vi "运维调试_采配水.vi"() -> ()   [LabVIEW 2016, in "PLC.lvlib"]
uses:
  PLC.lvlib
  control/switch.ctl
  <vilib>/Plasmionique/MB Master/MB_Master/MB_Master.lvclass
  <vilib>/Utility/miscctls.llb/LVPointTypeDef.ctl
  <vilib>/Plasmionique/MB Master/MB_Master_TCP/MB_Master_TCP.lvclass
  C:/Program Files (x86)/National Instruments/LabVIEW 2016/vi.lib/Plasmionique/MB Master/MB_Master/MB_Master.lvclass
  <vilib>/NI/Modbus Library/API/Wrapper/Create TCP Slave.vi
  <vilib>/NI/Modbus Library/API/slave/Modbus Slave.lvclass
  <vilib>/Plasmionique/MB Master/MB Master.lvlib
  <vilib>/NI/Modbus Library/API/Wrapper/API Main.lvlib
  <vilib>/Utility/config.llb/NI_LVConfig.lvlib
panel:
  in  "模拟量配置":bool
  out "过滤压力":sgl format="%#.4f"
  in  "三级过滤系统":bool
  out "配水泵计时":dbl
  out "氨氮水样池排液阀计时":dbl
  in  "M4":T1
  in  "V15":T1
  out "过滤出水阀计时":dbl
  out "过滤反冲洗阀计时":dbl
  out "过滤废水阀计时":dbl
  out "过滤回流阀计时":dbl
  out "过滤进样阀计时":dbl
  in  "V14-R":T1
  in  "V13-G":T1
  in  "V12":T1
  in  "V14-G":T1
  in  "V13-R":T1
  out "X8":bool caption="氨氮水样池液位开关_SL3"
  out "R122":i16 caption="氨氮水样池润洗时间"
  out "R123":i16 caption="过滤装置清洗时间"
  out "R121":i16 caption="过滤装置润洗时间"
  out "R120":i16 caption="加标回收配水时间"
  out "R116":i16 caption="储水时间设定"
  out "R115":i16 caption="清洗频次设定"
  out "R114":i16 caption="排液时间"
  out "R113":i16 caption="沉淀池清洗时间"
  out "R112":i16 caption="流通池清洗时间"
  out "R111":i16 caption="吹气时间"
  out "R110":i16 caption="外部管路清洗时间"
  out "R109":i16 caption="配水时间"
  out "R108":i16 caption="沉淀时间"
  out "R107":i16 caption="液位开关报警时间"
  out "R106":i16 caption="进样超时时间"
  out "R105":i16 caption="沉淀池润洗时间"
  out "R104":i16 caption="流通池润洗时间"
  out "沉淀池进样阀计时":dbl
  out "流通池进样阀计时":dbl
  in  "V3-R":T1
  in  "V3-G":T1
  out "状态":u16[](array[numeric])
  in  "更新程序":bool
  out "清洗次数":u16
  out "当前启动泵号":enum16{"1号泵", "2号泵"}(ring)
  in  "R117":u16(ring) caption="水箱储水水体" items=["自来水", "水样"]
  out "增压泵计时":dbl
  out "M2工作计时":dbl
  out "M1工作计时":dbl
  out "泵2反冲洗阀计时":dbl
  out "泵1反冲洗阀计时":dbl
  out "自来水出水阀计时":dbl
  out "进气阀计时":dbl
  out "流通池排液阀计时":dbl
  out "沉淀池排液阀计时":dbl
  out "沉淀池反冲洗阀计时":dbl
  out "流通池反冲洗阀计时":dbl
  out "泵2进样阀计时":dbl
  out "泵1进样阀计时":dbl
  in  "M3":T1
  in  "V11":T1
  in  "V10":T1
  in  "V2":T1
  in  "V1":T1
  in  "V7":T1
  in  "V6":T1
  out "X2":bool caption="进样水流开关_JY"
  out "采配水版本号":string
  out "通讯故障":bool
  in  "R102":u16(ring) caption="采水泵工作模式" items=["泵1单泵单管路", "泵2单泵单管路", "双泵双管路"]
  out "X7":bool caption="烟雾报警_YW"
  out "X6":bool caption="泵2过载报警_KM2"
  out "X5":bool caption="泵1过载报警_KM1"
  out "X4":bool caption="外部电源断电报警_DD1"
  out "X3":bool caption="水浸报警_SJ"
  out "X1":bool caption="沉淀池液位开关_YE2"
  out "X0":bool caption="流通池液位开关_YE1"
  out "集成报警信息":string
  out "R2":i16
  out "R1":i16
  out "多列列表框":i32(listbox)
  in  "V4":T1
  in  "V5":T1
  in  "V9":T1
  in  "V8":T1
  in  "M2":T1
  in  "M1":T1
  in  "返回":bool
  in  "参数设置":bool
  in  "单步启动":bool
  in  "启动":bool
  in  "停止":bool
  # "S"
  # "S"
  # "S"
  # "S"
  # "S"
  # "S"
  # "S"
  # "S"
  # "S"
  # "S"
  # "S"
  # "S"
  # "S"
  # "次"
  # "S"
  # "S"
  # "S"
  # "过滤压力："
  # "Mpa"
  # "单步计时："
  # "s"
  # "流程计时："
  # "s"
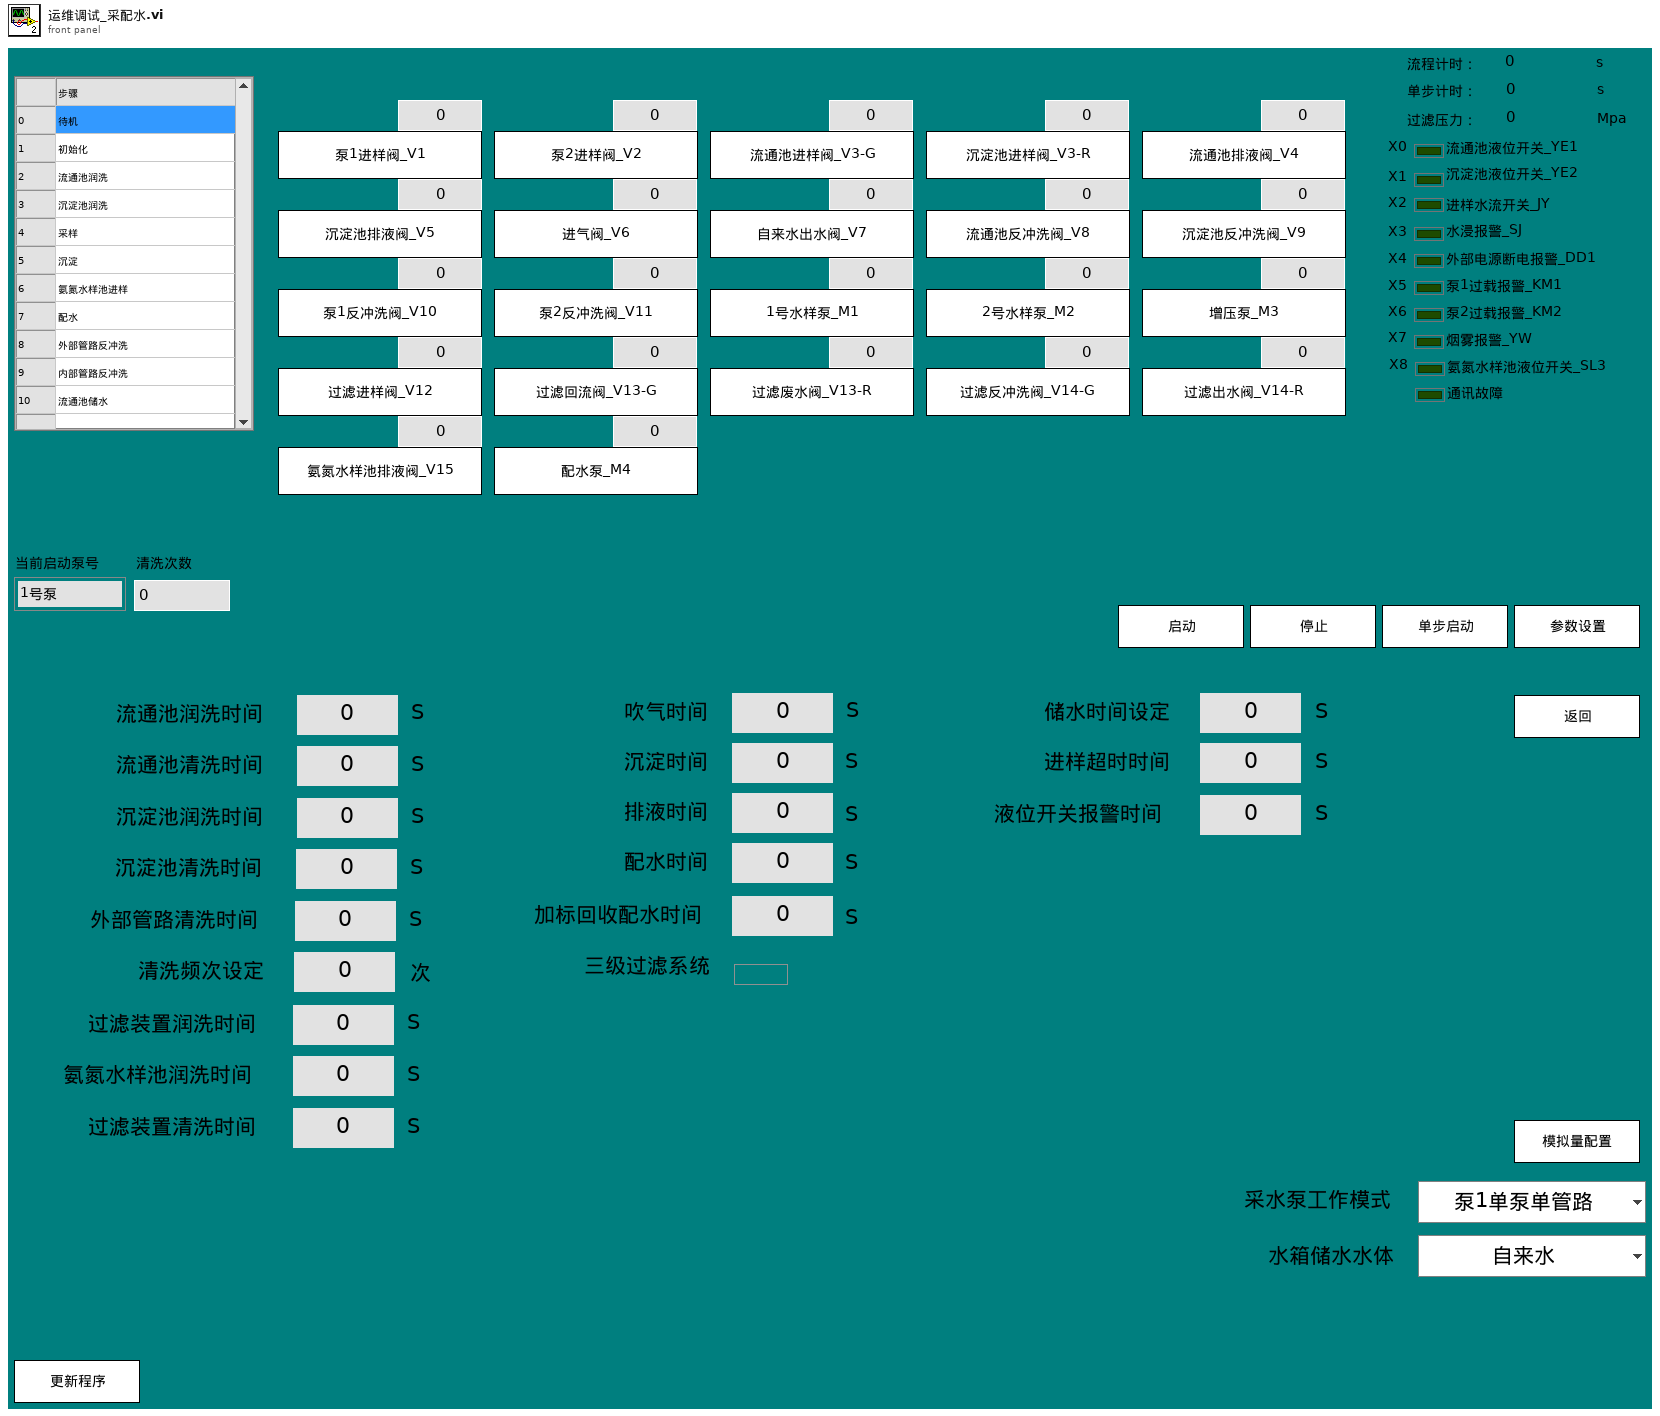
[diagram p1: front panel]
types:
  T1 = typedef "switch.ctl" = bool
  T2 = cluster{"R100":i16, "R101":i16, "R102":i16, "R103":i16, "R104":i16, "R105":i16, "R106":i16, "R107":i16, "R108":i16, "R109":i16, "R110":i16, "R111":i16, "R112":i16, "R113":i16, "R114":i16, "R115":i16, "R116":i16, "R117":i16, "R118":i16, "R119":i16, "R120":i16, "R121":i16, "R122":i16, "R123":i16}
  T3 = cluster{"R200":i16, "R201":i16, "R20 2":i16, "R20 3":i16, "R20 4":i16, "R20 5":i16, "R20 6":i16, "R20 7":i16, "R20 8":i16, "R20 9":i16, "R210":i16, "R211":i16, "R21 2":i16, "R21 3":i16, "R21 4":i16, "R21 5":i16, "R21 6":i16, "R21 7":i16, "R21 8":i16, "R21 9":i16, "R220":i16, "R221":i16, "R22 2":i16, "R22 3":i16, "R22 4":i16, "R22 5":i16, "R22 6":i16, "R22 7":i16, "R22 8":i16, "R22 9":i16, "R230":i16, "R231":i16}
  T4 = typedef "LVPointTypeDef.ctl" = cluster{"Horizontal":i16, "Vertical":i16}
  T5 = typedef "NI_LVConfig.lvlib/Config Data RefNum.ctl" = refnum<k1>
  T6 = cluster{"时间标识":timestamp, "设备":string, "日志信息":string}
  T7 = cluster{"R0":i16, "R1":i16, "R2":i16, "R3":i16, "R4":i16, "R5":i16, "R6":i16, "R7":i16, "R8":i16, "R9":i16, "R10":i16, "R11":i16, "R12":i16, "R13":i16, "R14":i16, "R15":i16, "R16":i16, "R17":i16, "R18":i16, "R19":i16, "R20":i16, "R21":i16, "R22":i16, "R23":i16, "R24":i16, "R25":i16, "R26":i16, "R27":i16, "R28":i16, "R29":i16, "R30":i16, "R31":i16, "R32":i16, "R33":i16, "R34":i16, "R35":i16, "R36":i16, "R37":i16, "R38":i16, "R39":i16}
  T8 = cluster{"seconds since 1Jan1904":timestamp, "table输入":string, string, "table输入":string}
  T9 = cluster{"时间标识":timestamp, "设备":string, "日志信息":string, "流程参数":string}
  T10 = cluster{"命令":string, cluster{"starting address":u16, "holding register value":u16}}
  T11 = cluster{"命令":string, "数据":cluster{"starting address":u16, "holding register value":u16}}
  T12 = cluster{"命令":string, "数据":cluster{"starting address":u16, "holding register values":u16[]}}
  T13 = cluster{"命令":string, "data":cluster{"starting address":u16, "coil values":bool[]}}
  T14 = cluster{"参数启用":cluster{"氨氮":bool, "总磷":bool, "总氮":bool, "多参数":bool, "CODMn":bool, "CODcr":bool, "超标留样":bool}}
  T15 = enum32{"Bad", "Idle", "Run top level", "Running"}
  T16 = cluster{"starting address":u16, "holding register values":u16[]}
  T17 = cluster{"starting address":u16, "holding register value":u16}
  T18 = cluster{"starting address":u16, "coil values":bool[]}
  T19 = cluster{"Registers[0]":u16, "Registers[1]":u16, "Registers[2]":u16, "Registers[3]":u16, "Registers[4]":u16, "Registers[5]":u16, "Registers[6]":u16, "Registers[7]":u16, "Registers[8]":u16, "Registers[9]":u16, "Registers[10]":u16, "Registers[11]":u16, "Registers[12]":u16, "Registers[13]":u16, "Registers[14]":u16, "Registers[15]":u16, "Registers[16]":u16, "Registers[17]":u16, "Registers[18]":u16, "Registers[19]":u16, "Registers[20]":u16, "Registers[21]":u16, "Registers[22]":u16, "Registers[23]":u16, "Registers[24]":u16, "Registers[25]":u16, "Registers[26]":u16, "Registers[27]":u16, "Registers[28]":u16, "Registers[29]":u16, "Registers[30]":u16, "Registers[31]":u16, "Registers[32]":u16, "Registers[33]":u16, "Registers[34]":u16, "Registers[35]":u16, "Registers[36]":u16, "Registers[37]":u16, "Registers[38]":u16, "Registers[39]":u16}
  T20 = cluster{"Registers[0]":u16, "Registers[1]":u16, "Registers[2]":u16, "Registers[3]":u16, "Registers[4]":u16, "Registers[5]":u16, "Registers[6]":u16, "Registers[7]":u16, "Registers[8]":u16, "Registers[9]":u16, "Registers[10]":u16, "Registers[11]":u16, "Registers[12]":u16, "Registers[13]":u16, "Registers[14]":u16, "Registers[15]":u16, "Registers[16]":u16, "Registers[17]":u16, "Registers[18]":u16, "Registers[19]":u16, "Registers[20]":u16, "Registers[21]":u16, "Registers[22]":u16, "Registers[23]":u16, "Registers[24]":u16, "Registers[25]":u16, "Registers[26]":u16, "Registers[27]":u16, "Registers[28]":u16, "Registers[29]":u16, "Registers[30]":u16, "Registers[31]":u16}
  T21 = cluster{"Registers[0]":u16, "Registers[1]":u16, "Registers[2]":u16, "Registers[3]":u16, "Registers[4]":u16, "Registers[5]":u16}
  T22 = cluster{"X0":dbl, "X1":dbl, "Y0":dbl, "Y1":dbl}[]
  T23 = cluster{"[0]":dbl, "[1]":dbl, "[2]":dbl, "[3]":dbl, "[4]":dbl, "[5]":dbl}
  T24 = cluster{"Registers[0]":u16, "Registers[1]":u16, "Registers[2]":u16, "Registers[3]":u16, "Registers[4]":u16, "Registers[5]":u16, "Registers[6]":u16, "Registers[7]":u16, "Registers[8]":u16, "Registers[9]":u16, "Registers[10]":u16, "Registers[11]":u16, "Registers[12]":u16, "Registers[13]":u16, "Registers[14]":u16, "Registers[15]":u16, "Registers[16]":u16, "Registers[17]":u16, "Registers[18]":u16, "Registers[19]":u16, "Registers[20]":u16, "Registers[21]":u16, "Registers[22]":u16, "Registers[23]":u16}
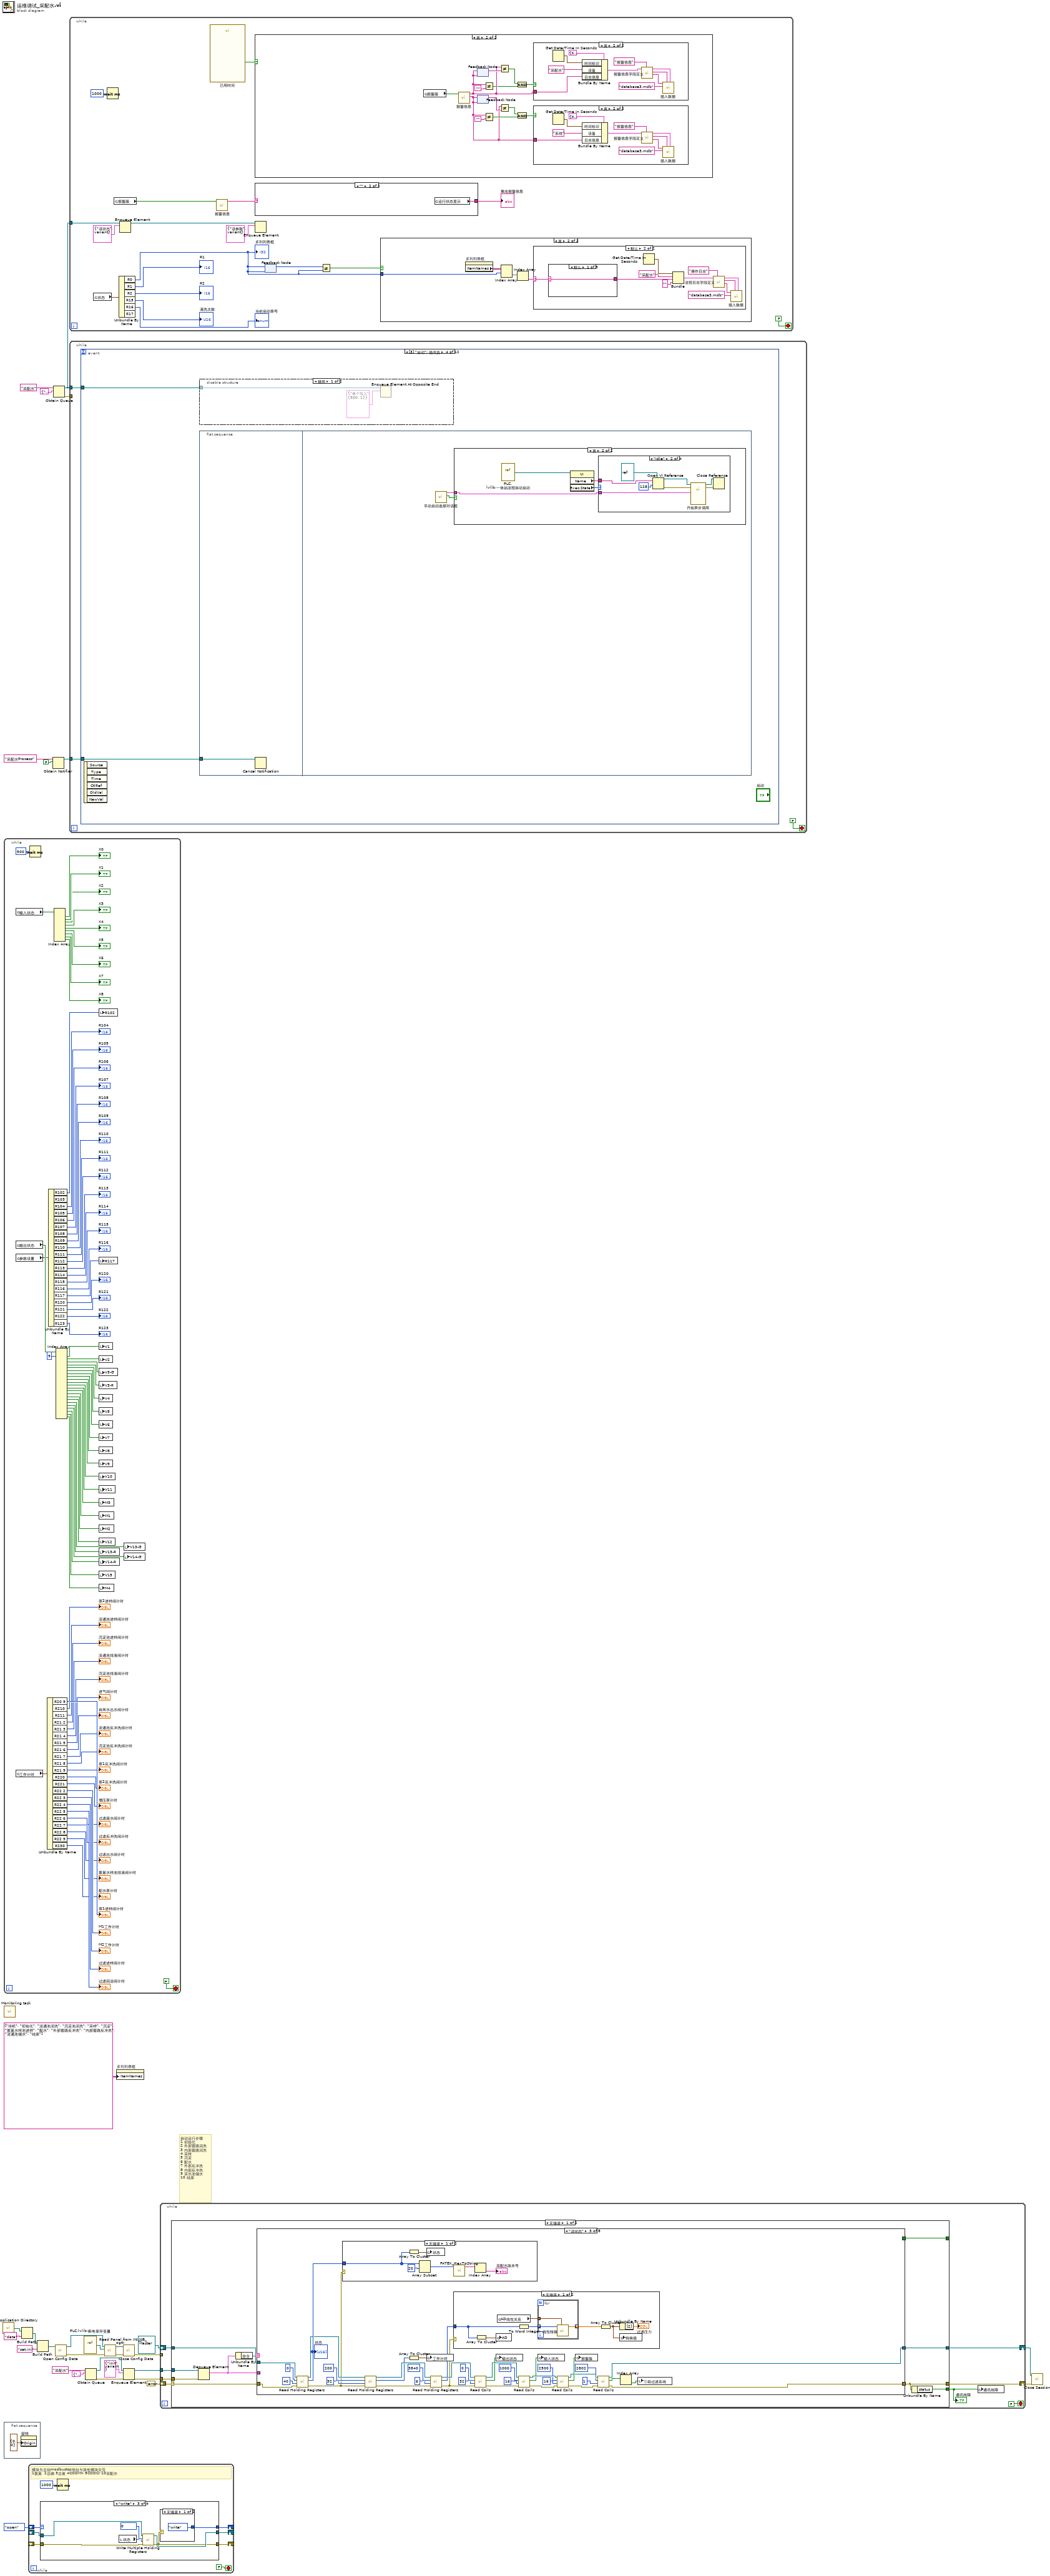
[diagram p0: block diagram]
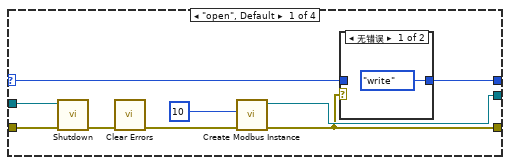
[diagram p2: hidden frame]
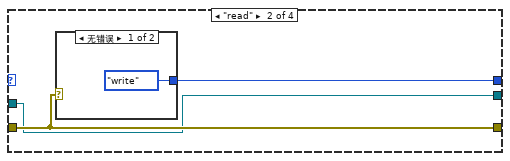
[diagram p4: hidden frame]
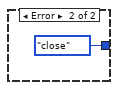
[diagram p5: hidden frame]
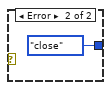
[diagram p6: hidden frame]
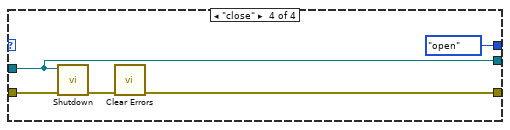
[diagram p7: hidden frame]
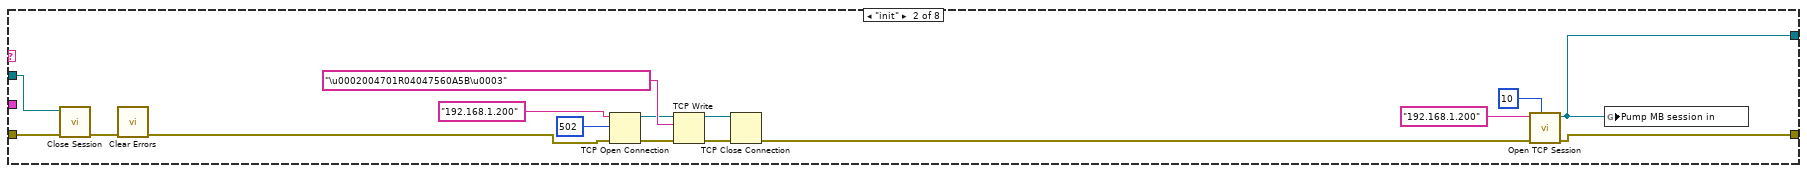
[diagram p9: hidden frame]
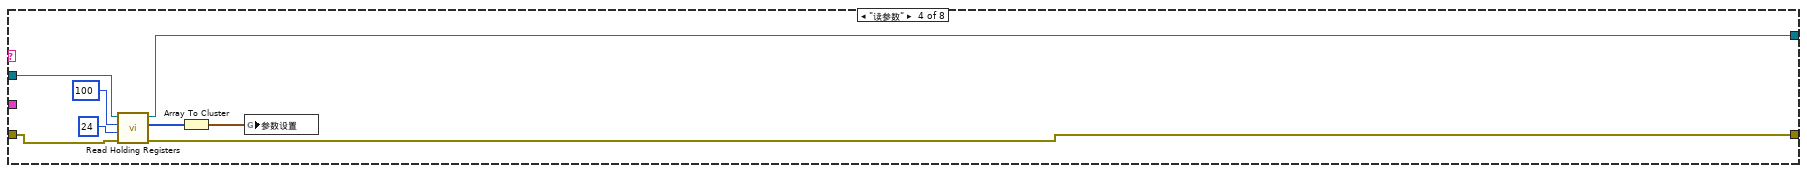
[diagram p12: hidden frame]
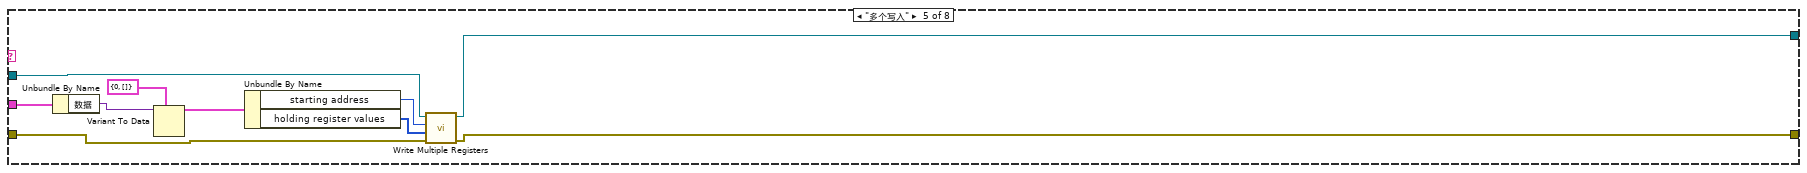
[diagram p13: hidden frame]
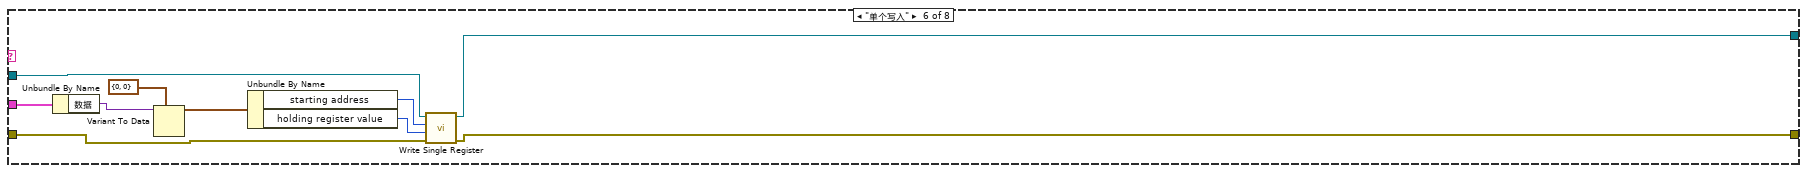
[diagram p14: hidden frame]
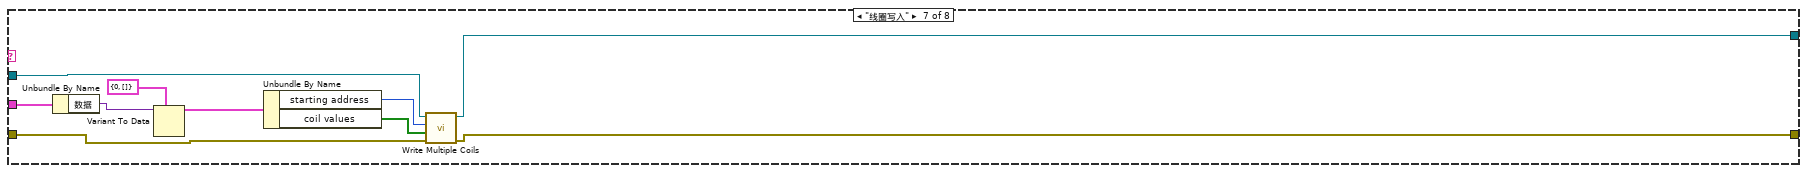
[diagram p15: hidden frame]
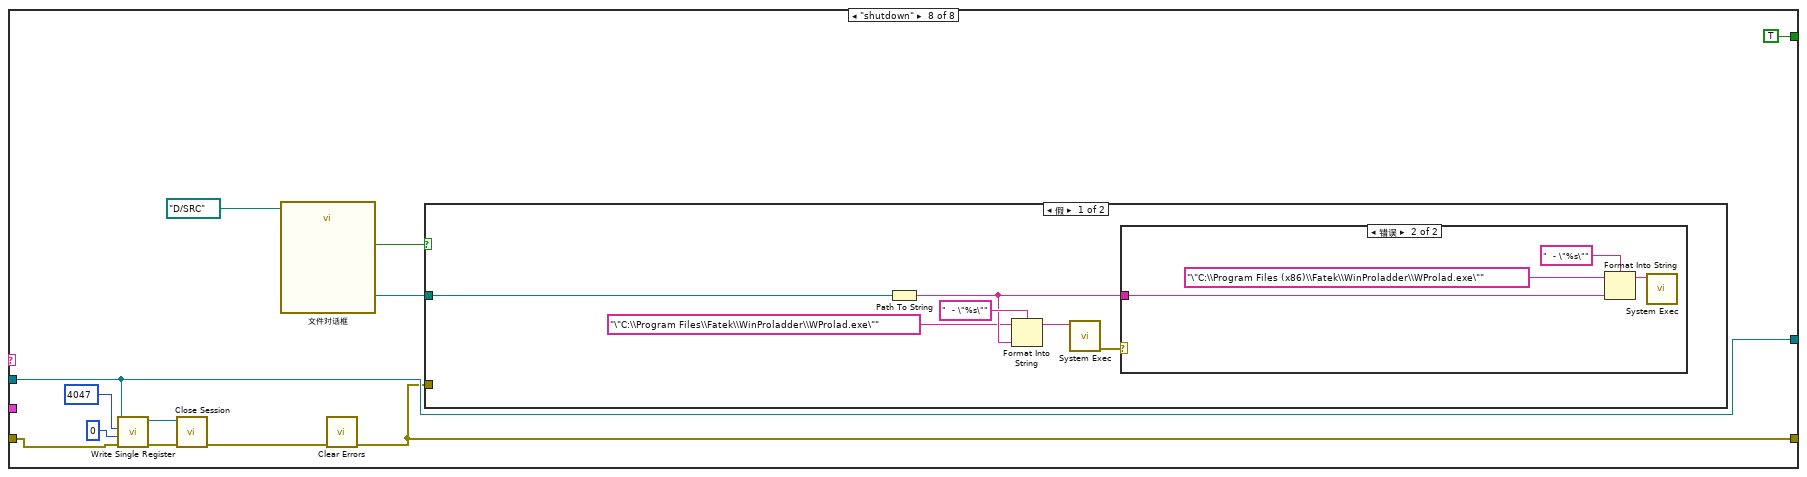
[diagram p16: hidden frame]
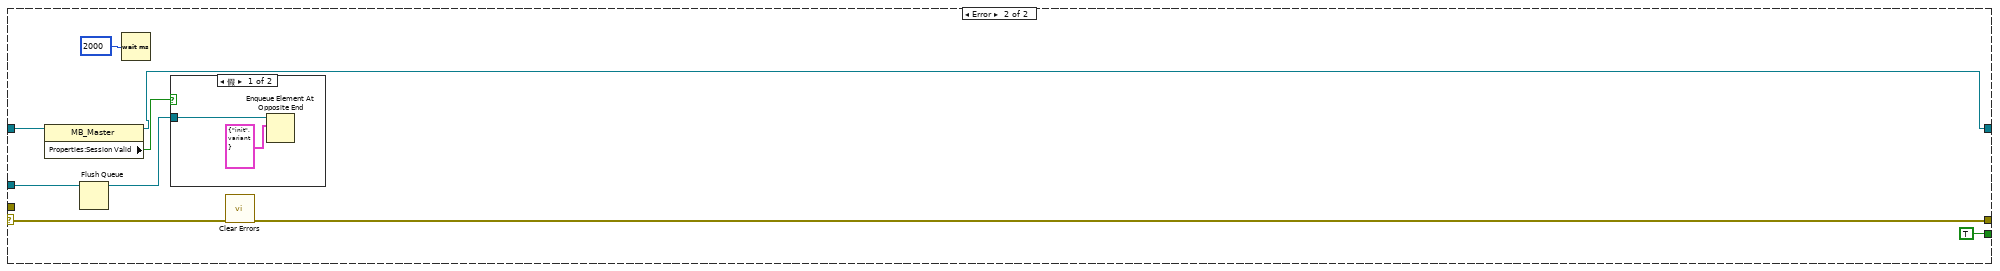
[diagram p19: hidden frame]
diagram:
  # "自动运行步骤\n1 初始化\n2 外部管路润洗\n3 内部管路润洗\n4 采样\n5 沉淀\n6 配水\n7 外部反冲洗\n8 内部反冲洗\n9 采水池储水\n10 结束"
  n1 = call <vilib>:"Application Directory.vi"() -> ("Application Directory"=w3:path)
  n2 = while {
    stop <- FALSE stop-if-true
    n3 = global read "采配水全局变量.vi" "输入状态"() -> (w93:bool[])
    n4 = global read "采配水全局变量.vi" "输出状态"() -> (w109:bool[])
    n5 = global read "采配水全局变量.vi" "参数设置"() -> (w66:T2)
    n6 = global read "采配水全局变量.vi" "工作计时"() -> (w82:T3)
    n7 = Wait (ms)(milliseconds to wait=u32 500 ("等待时间（毫秒）")) -> ()  [unwired: 1 out]
    n8 = Unbundle By Name(w82) -> ("R20 9"=→"泵1进样阀计时":i16, "R210"=→"泵2进样阀计时":i16, "R211"=→"流通池进样阀计时":i16, "R21 2"=→"沉淀池进样阀计时":i16, "R21 3"=→"流通池排液阀计时":i16, "R21 4"=→"沉淀池排液阀计时":i16, "R21 5"=→"进气阀计时":i16, "R21 6"=→"自来水出水阀计时":i16, "R21 7"=→"流通池反冲洗阀计时":i16, "R21 8"=→"沉淀池反冲洗阀计时":i16, "R21 9"=→"泵1反冲洗阀计时":i16, "R220"=→"泵2反冲洗阀计时":i16, "R221"=→"增压泵计时":i16, "R22 2"=→"M1工作计时":i16, "R22 3"=→"M2工作计时":i16, "R22 4"=→"过滤进样阀计时":i16, "R22 5"=→"过滤回流阀计时":i16, "R22 6"=→"过滤废水阀计时":i16, "R22 7"=→"过滤反冲洗阀计时":i16, "R22 8"=→"过滤出水阀计时":i16, "R22 9"=→"氨氮水样池排液阀计时":i16, "R230"=→"配水泵计时":i16)
    n9 = Unbundle By Name(w66) -> ("R102"=w65:i16, "R104"=→"R104":i16, "R105"=→"R105":i16, "R106"=→"R106":i16, "R107"=→"R107":i16, "R108"=→"R108":i16, "R109"=→"R109":i16, "R110"=→"R110":i16, "R111"=→"R111":i16, "R112"=→"R112":i16, "R113"=→"R113":i16, "R114"=→"R114":i16, "R115"=→"R115":i16, "R116"=→"R116":i16, "R117"=w51:i16, "R120"=→"R120":i16, "R121"=→"R121":i16, "R122"=→"R122":i16, "R123"=→"R123":i16)  [unwired: 1 out]
    n10 = Index Array(array=w93) -> (element #1=→"X0":bool, element #2=→"X1":bool, element #3=→"X2":bool, element #4=→"X3":bool, element #5=→"X4":bool, element #6=→"X5":bool, element #7=→"X6":bool, element #8=→"X7":bool, element #9=→"X8":bool)  [unwired: 9 in]
    n11 = Index Array(array=w109, index #1=9 ("索引")) -> (element #1=w107:bool, element #2=w106:bool, element #3=w105:bool, element #4=w104:bool, element #5=w103:bool, element #6=w102:bool, element #7=w101:bool, element #8=w100:bool, element #9=w83:bool, element #10=w84:bool, element #11=w99:bool, element #12=w98:bool, element #13=w97:bool, element #14=w96:bool, element #15=w95:bool, element #16=w47:bool, element #17=w46:bool, element #18=w45:bool, element #19=w44:bool, element #20=w43:bool, element #21=w42:bool, element #22=w41:bool)  [unwired: 21 in]
    n12 = local write "R102"(w65) -> ()
    n13 = local write "R117"(w51) -> ()
    n14 = local write "V1"(w107) -> ()
    n15 = local write "V2"(w106) -> ()
    n16 = local write "V3-G"(w105) -> ()
    n17 = local write "V3-R"(w104) -> ()
    n18 = local write "V4"(w103) -> ()
    n19 = local write "V5"(w102) -> ()
    n20 = local write "V6"(w101) -> ()
    n21 = local write "V7"(w100) -> ()
    n22 = local write "V8"(w83) -> ()
    n23 = local write "V9"(w84) -> ()
    n24 = local write "V10"(w99) -> ()
    n25 = local write "V11"(w98) -> ()
    n26 = local write "M3"(w97) -> ()
    n27 = local write "M1"(w96) -> ()
    n28 = local write "M2"(w95) -> ()
    n29 = local write "V12"(w47) -> ()
    n30 = local write "V13-R"(w45) -> ()
    n31 = local write "V14-R"(w43) -> ()
    n32 = local write "V15"(w42) -> ()
    n33 = local write "M4"(w41) -> ()
    n34 = local write "V13-G"(w46) -> ()
    n35 = local write "V14-G"(w44) -> ()
  }
  n36 = call "Monitoring task.vi"() -> ()  [unwired: 12 in]
  n37 = flat-sequence {
    frame #0 {
      n38 = property on="窗格" class="Pane"("Origin"=T4 {"Horizontal"=0, "Vertical"=0} ("原点")) -> ()  [unwired: 2 in, 2 out]
    }
  }
  n39 = Build Path(base path=w3, name or relative path="data" ("名称或相对路径")) -> (appended path=w5:path)
  n40 = while {
    shift-right: [w117] -> _
    shift-left: _ -> [w119]
    shift-right: [w116] -> _
    shift-left: _ -> [w118]
    shift-right: [w113] -> _
    shift-left: enum16{"open", "read", "write", "close"}."open" -> [w114]
    stop <- FALSE stop-if-true
    # "模块为主站modbustcp地址与其他模块交互\n1氨氮  2总磷 3总氮 4CODMn 5CODCr 10采配水"
    n41 = case shown="\"write\"" w114 {
      selector: w114 -> [w128 _ _ _]
      tunnel: w119 -> [w122 w131 w141 w147]
      tunnel: w118 -> [w121 w132 w140 w146]
      tunnel: [w125 w131 w138 w147] -> w117
      tunnel: [w124 w132 w137 w149] -> w116
      tunnel: [w127 w133 w142 enum16{"open", "read", "write", "close"}."open"] -> w113
      frame "open", Default {
        n42 = call-dynamic "Shutdown.vi"("error in"=w121, "Modbus slave in"=w122) -> ("error out"=w120:errorcluster)  [unwired: 9 in]
        n43 = call <vilib>:"Clear Errors.vi"("error in (no error)"=w120) -> ("error out"=w123:errorcluster)  [unwired: 5 in, 1 out]
        n44 = call-poly <vilib>:"Create Modbus Instance.vi"("error in"=w123, "port (502)"=u16 10) -> ("error out"=w124:errorcluster, "TCP slave instance"=w125:refnum<class "Modbus Slave.lvclass">)  [unwired: 8 in]
        n45 = case shown="无错误" w124 {
          tunnel: w128 -> [_ w130]
          tunnel: [enum16{"open", "read", "write", "close"}."write" w130] -> w127
          frame No Error {
          }
          frame Error {
          }
        }
      }
      frame "read" {
        n46 = case shown="无错误" w132 {
          tunnel: [enum16{"open", "read", "write", "close"}."write" enum16{"open", "read", "write", "close"}."close"] -> w133
          frame No Error {
          }
          frame Error {
          }
        }
      }
      frame "write" {
        n47 = local read "状态"() -> (w136:u16[])
        n48 = call-dynamic "Write Multiple Holding Registers.vi"("error in"=w140, "registers to write"=w136, "starting address"=u16 0, "Modbus slave in"=w141) -> ("error out"=w137:errorcluster, "Modbus slave out"=w138:refnum<class "Modbus Slave.lvclass">)  [unwired: 6 in]
        n49 = case shown="无错误" w137 {
          tunnel: [enum16{"open", "read", "write", "close"}."write" enum16{"open", "read", "write", "close"}."close"] -> w142
          frame No Error {
          }
          frame Error {
          }
        }
      }
      frame "close" {
        n50 = call-dynamic "Shutdown.vi"("error in"=w146, "Modbus slave in"=w147) -> ("error out"=w145:errorcluster)  [unwired: 9 in]
        n51 = call <vilib>:"Clear Errors.vi"("error in (no error)"=w145) -> ("error out"=w149:errorcluster)  [unwired: 5 in, 1 out]
      }
    }
    n52 = Wait (ms)(milliseconds to wait=u32 1000 ("等待时间（毫秒）")) -> ()  [unwired: 1 out]
  }
  n53 = Build Path(base path=w5, name or relative path="set.ini" ("名称或相对路径")) -> (appended path=w7:path)
  n54 = Obtain Notifier(name (unnamed)="采配水Process" ("名称（未命名）"), notification data type=FALSE) -> (notifier out=w24:refnum<notifier>)  [unwired: 2 in, 2 out]
  n55 = Obtain Queue(name (unnamed)="采配水" ("名称（未命名）"), element data type=cluster{"命令":string, "数据":variant} {"命令"="", "数据"=variant}) -> (queue out=w28:refnum<queue>, error out=w29:errorcluster)  [unwired: 3 in, 1 out]
  n56 = call <vilib>:"Open Config Data.vi"("configuration file path"=w7) -> ("error out"=w8:errorcluster, "refnum"=w2:T5)  [unwired: 8 in, 1 out]
  n57 = while {
    tunnel: w28 -> [w166]
    stop <- FALSE stop-if-true
    n58 = global read "采配水全局变量.vi" "状态"() -> (w164:T7)
    n59 = Wait (ms)(milliseconds to wait=u32 1000 ("等待时间（毫秒）")) -> ()  [unwired: 1 out]
    n60 = global read "采配水全局变量.vi" "报警簇"() -> (w160:bool[])
    n61 = Unbundle By Name(w164) -> ("R0"=w153:i16, "R1"=→"R1":i16, "R2"=→"R2":i16, "R15"=→"清洗次数":i16, "R16"=→"当前启动泵号":i16)  [unwired: 1 out]
    "多列列表框" <- w153
    n62 = Enqueue Element(queue=w166, element=cluster{"命令":string, "数据":variant} {"命令"="读状态", "数据"=variant} ("元素")) -> (queue out=w155:refnum<queue>)  [unwired: 2 in, 2 out]
    n63 = call "已用时间"() -> ("Time has Elapsed"=w158:bool)  [unwired: 12 in, 7 out]
    n64 = call "报警信息.vi"("报警簇"=w160) -> ("采配水报警信息"=w152:string)  [unwired: 9 in, 1 out]
    n65 = case shown="真" w158 {
      frame False {
      }
      frame True {
        n66 = global read "采配水全局变量.vi" "报警簇"() -> (w180:bool[])
        n67 = call "报警信息.vi"("报警簇"=w180) -> ("系统报警信息"=w169:string, "采配水报警信息"=w176:string)  [unwired: 9 in]
        n68 = feedback #1(w176) -> (w179:string)
        n69 = feedback-in #1(w176) -> ()
        n70 = feedback #2(w169) -> (w170:string)
        n71 = feedback-in #2(w169) -> ()
        n72 = Not Equal?(x=w176, y="") -> (x != y?=w174:bool)
        n73 = Not Equal?(x=w169, y="") -> (x != y?=w173:bool)
        n74 = Not Equal?(x=w176, y=w179) -> (x != y?=w178:bool)
        n75 = Not Equal?(x=w169, y=w170) -> (x != y?=w171:bool)
        n76 = And(x=w178, y=w174) -> (x .and. y?=w177:bool)
        n77 = And(x=w171, y=w173) -> (x .and. y?=w168:bool)
        n78 = case shown="真" w177 {
          tunnel: w176 -> [_ w191]
          frame False {
          }
          frame True {
            n79 = Get Date/Time In Seconds() -> (seconds since 1Jan1904=w193:timestamp)
            n80 = Bundle By Name(cluster=T6 {"时间标识"=timestamp(0 s since 1904-01-01), "设备"="", "日志信息"=""} ("data in"), "时间标识"=w193, "设备"="采配水", "日志信息"=w191) -> (w194:T6)
            n81 = call "报警信息字段定义.vi"("table输入"="报警信息", "data in"=w194) -> ("table输出"=w198:string, "columns"=w199:string[], "data out"=w200:T6)  [unwired: 7 in]
            n82 = call "插入数据.vi"("data"=w200, "columns"=w199, "database"="database3.mdb", "table"=w198) -> ()  [unwired: 7 in, 1 out]
          }
        }
        n83 = case shown="真" w168 {
          tunnel: w169 -> [_ w181]
          frame False {
          }
          frame True {
            n84 = Get Date/Time In Seconds() -> (seconds since 1Jan1904=w183:timestamp)
            n85 = Bundle By Name(cluster=T6 {"时间标识"=timestamp(0 s since 1904-01-01), "设备"="", "日志信息"=""} ("data in"), "时间标识"=w183, "设备"="系统", "日志信息"=w181) -> (w184:T6)
            n86 = call "报警信息字段定义.vi"("table输入"="报警信息", "data in"=w184) -> ("table输出"=w188:string, "columns"=w189:string[], "data out"=w190:T6)  [unwired: 7 in]
            n87 = call "插入数据.vi"("data"=w190, "columns"=w189, "database"="database3.mdb", "table"=w188) -> ()  [unwired: 7 in, 1 out]
          }
        }
      }
    }
    n88 = case shown="\"\"" w152 {
      selector: w152 -> [w201 _]
      tunnel: [w201 w202] -> w159
      frame Default {
      }
      frame "" {
        n89 = global read "采配水全局变量.vi" "运行状态显示"() -> (w202:string)
      }
    }
    "集成报警信息" <- w159
    n90 = Enqueue Element(queue=w155, element=cluster{"命令":string, "数据":variant} {"命令"="读参数", "数据"=variant} ("元素")) -> ()  [unwired: 2 in, 3 out]
    n91 = feedback-in #3(w153) -> ()
    n92 = feedback #3(w153) -> (w154:i16)
    n93 = Not Equal?(x=w154, y=w153) -> (x != y?=w161:bool)
    n94 = case shown="真" w161 {
      tunnel: w153 -> [_ w205]
      frame False {
      }
      frame True {
        n95 = property on="多列列表框" class="MCListbox (严格)"() -> ("ItemNames"=w206:string[][])  [unwired: 2 in, 2 out]
        n96 = Index Array(array=w206, index (row)=w205) -> (element=w204:string[])  [unwired: 1 in]
        n97 = Index Array(array=w204) -> (element=w203:string)  [unwired: 1 in]
        n98 = case shown="默认" w203 {
          selector: w203 -> [_ w208]
          frame "待机" {
          }
          frame Default {
            n99 = case shown="默认" w208 {
              selector: w208 -> [w218 _ _]
              tunnel: [w218 "-->>启动" "-->>结束"] -> w207
              frame Default {
              }
              frame "初始化" {
              }
              frame "结束" {
              }
            }
            n100 = Get Date/Time In Seconds() -> (seconds since 1Jan1904=w212:timestamp)
            n101 = Bundle("seconds since 1Jan1904"=w212, "table输入"="采配水", w207, "table输入"="") -> (w210:T8)  [unwired: 1 in]
            n102 = call "流程日志字段定义.vi"("table输入"="操作日志", "data in"=w210) -> ("table输出"=w215:string, "columns"=w216:string[], "data out"=w217:T9)  [unwired: 7 in]
            n103 = call "插入数据.vi"("data"=w217, "columns"=w216, "database"="database3.mdb", "table"=w215) -> ()  [unwired: 7 in, 1 out]
          }
        }
      }
    }
  }
  n104 = while {
    tunnel: w28 -> [w222]
    tunnel: w29 -> [_]
    tunnel: w24 -> [w221]
    stop <- FALSE stop-if-true
    n105 = event shown="[3] \"启动\": 值改变" {
      selector: _ -> [_ _ _ _ _ _ _ _ _ _ _ _]
      dyn-events: _ -> [_ _ _ _ _ _ _ _ _ _ _ _]
      timeout: _ -> [_ _ _ _ _ _ _ _ _ _ _ _]
      tunnel: w222 -> [_ _ w226 w229 w251 w259 _ _ _ w315 w318 w325]
      tunnel: w221 -> [_ _ w225 w228 _ _ _ _ _ _ _ _]
      event Timeout {
        n106 = event-data() -> ()  [unwired: 1 in, 3 out]
      }
      event "模拟量配置": Value Change {
        n107 = event-data() -> ()  [unwired: 1 in, 6 out]
        n108 = call "模拟量设置窗口.vi"() -> ()  [unwired: 12 in]
      }
      event "停止": Value Change {
        n109 = event-data() -> ()  [unwired: 1 in, 6 out]
        n110 = Send Notification(notification=TRUE ("通知"), notifier=w225) -> ()  [unwired: 1 in, 2 out]
        n111 = Enqueue Element At Opposite End(queue=w226, element=T10 {"命令"="单个写入", {"starting address"=300, "holding register value"=2}} ("元素")) -> ()  [unwired: 2 in, 3 out]
      }
      event "启动": Value Change {
        n112 = event-data() -> ()  [unwired: 1 in, 6 out]
        n113 = disable-structure shown="禁用" {
          disable-tunnel: w229 -> [w247 _]
          frame Disabled {
            n114 = Enqueue Element At Opposite End(queue=w247, element=T10 {"命令"="单个写入", {"starting address"=300, "holding register value"=1}} ("元素")) -> ()  [unwired: 2 in, 3 out]
          }
          frame Enabled {
          }
        }
        n115 = flat-sequence {
          tunnel: w228 -> [w230]
          frame #0 {
            n116 = Cancel Notification(0:w230) -> ()  [unwired: 1 in, 3 out]
          }
          frame #1 {
            n117 = call "手动启动选择对话框.vi"() -> ("确定"=w232:bool, "输出簇"=w231:T14)  [unwired: 10 in]
            n118 = case shown="真" w232 {
              tunnel: w231 -> [_ w233]
              frame False {
              }
              frame True {
                n119 = vi-ref "PLC.lvlib:一体站流程自动启动.vi"() -> (w236:refnum<vi>)
                n120 = property class="VI"(reference=w236) -> ("Name"=w235:string, "Exec.State"=w234:T15)  [unwired: 1 in, 2 out]
                n121 = case shown="\"Idle\"" w234 {
                  tunnel: w235 -> [_ w244 _ _]
                  tunnel: w233 -> [_ w238 _ _]
                  frame "Bad", Default {
                  }
                  frame "Idle" {
                    n122 = Open VI Reference(type specifier VI Refnum (for type only)=refnum<vi> refnum, vi path=w244, options=128 ("选项")) -> (vi reference=w242:refnum<vi>, error out=w240:errorcluster)  [unwired: 3 in]
                    n123 = call-by-ref "开始异步调用"(reference=w242, error in=w240, "参数"=w238) -> (reference out=w241:refnum<vi>, error out=w239:errorcluster)  [unwired: 11 in]
                    n124 = Close Reference(reference=w241, error in (no error)=w239) -> ()  [unwired: 1 out]
                  }
                  frame "Run top level" {
                  }
                  frame "Running" {
                    n125 = One Button Dialog(message="流程已启动，无需重复启动！" ("消息")) -> ()  [unwired: 1 in, 1 out]
                  }
                }
              }
            }
          }
        }
      }
      event "单步启动": Value Change {
        n126 = event-data() -> ()  [unwired: 1 in, 6 out]
        n127 = call "单步启动对话框.vi"() -> ("单步启动步骤输出"=w248:u16)  [unwired: 11 in]
        n128 = Bundle By Name(cluster=T11 {"命令"="单个写入", "数据"={"starting address"=301, "holding register value"=0}} ("元素"), "数据.holding register value"=w248) -> (w249:T11)
        n129 = Enqueue Element At Opposite End(queue=w251, element=w249) -> ()  [unwired: 2 in, 3 out]
      }
      event "R104", "R117", "R105", "R106", "R107", "R108", "R109", "R110", "R111", "R112", "R113", "R114", "R115", "R116", "R102", "R120", "R121", "R123", "R122": Value Change {
        n130 = event-data() -> ()  [unwired: 1 in, 6 out]
        n131 = local read "R104"() -> (w277:i16)
        n132 = local read "R105"() -> (w276:i16)
        n133 = local read "R106"() -> (w275:i16)
        n134 = local read "R107"() -> (w274:i16)
        n135 = local read "R108"() -> (w273:i16)
        n136 = local read "R109"() -> (w272:i16)
        n137 = local read "R110"() -> (w271:i16)
        n138 = local read "R111"() -> (w270:i16)
        n139 = local read "R112"() -> (w269:i16)
        n140 = local read "R113"() -> (w268:i16)
        n141 = local read "R114"() -> (w267:i16)
        n142 = local read "R115"() -> (w266:i16)
        n143 = local read "R116"() -> (w265:i16)
        n144 = Build Array("R102", u16 0 ("元素"), w277, w276, w275, w274, w273, w272, w271, w270, w269, w268, w267, w266, w265, "R117") -> (w278:u16[])
        n145 = local read "R120"() -> (w257:i16)
        n146 = local read "R121"() -> (w255:i16)
        n147 = local read "R122"() -> (w254:i16)
        n148 = local read "R123"() -> (w253:i16)
        n149 = Build Array(w257, w255, w254, w253) -> (w256:i16[])
        n150 = Bundle By Name(cluster=T12 {"命令"="多个写入", "数据"={"starting address"=0, "holding register values"=[]}} ("元素"), "数据.starting address"=u16 102, "数据.holding register values"=w278) -> (w280:T12)
        n151 = Flush Queue(queue=w259) -> (queue out=w252:refnum<queue>)  [unwired: 1 in, 2 out]
        n152 = Bundle By Name(cluster=T12 {"命令"="多个写入", "数据"={"starting address"=0, "holding register values"=[]}} ("元素"), "数据.starting address"=u16 120, "数据.holding register values"=w256) -> (w262:T12)
        n153 = Enqueue Element At Opposite End(queue=w252, element=w280) -> (error out=w258:errorcluster)  [unwired: 2 in, 2 out]
        n154 = Enqueue Element At Opposite End(queue=w252, element=w262, error in (no error)=w258) -> ()  [unwired: 1 in, 3 out]
      }
      event "R104", "R105", "R106", "R107", "R108", "R109", "R110", "R111", "R112", "R113", "R114", "R115", "R116", "R120", "R122", "R123", "R121": Mouse Down {
        n155 = event-data() -> ("CtlRef"=w286:refnum<vi>)  [unwired: 1 in, 7 out]
        n156 = property class="DigNum (严格)"(reference=w286) -> (reference out=w284:refnum<vi>, "Value"=w285:i16)  [unwired: 1 in, 1 out]
        n157 = call "数字键盘.vi"("OldNumber"=w285) -> ("NewNumber"=w283:sgl)
        n158 = property class="DigNum (严格)"(reference=w284, "Val(Sgnl)"=w283) -> ()  [unwired: 1 in, 2 out]
      }
      event "参数设置": Value Change {
        n159 = event-data() -> ()  [unwired: 1 in, 6 out]
        n160 = property on="窗格" class="Pane"("Origin"=T4 {"Horizontal"=0, "Vertical"=628} ("原点")) -> ()  [unwired: 2 in, 2 out]
      }
      event "返回": Value Change {
        n161 = event-data() -> ()  [unwired: 1 in, 6 out]
        n162 = property on="窗格" class="Pane"("Origin"=T4 {"Horizontal"=0, "Vertical"=0} ("原点")) -> ()  [unwired: 2 in, 2 out]
      }
      event Value Change {
        n163 = event-data() -> ()  [unwired: 1 in, 6 out]
        n164 = Build Array("V1", "V2", "V3-G", "V3-R", "V4", "V5", "V6", "V7", "V8", "V9", "V10", "V11", "M3", "M1", "M2", "V12", "V13-G", "V13-R", "V14-G", "V14-R", "V15", "M4") -> (w312:T1[])
        n165 = Bundle By Name(cluster=T13 {"命令"="线圈写入", "data"={"starting address"=2409, "coil values"=[]}} ("元素"), "data.coil values"=w312) -> (w313:T13)
        n166 = Flush Queue(queue=w315) -> (queue out=w289:refnum<queue>)  [unwired: 1 in, 2 out]
        n167 = Enqueue Element At Opposite End(queue=w289, element=w313) -> ()  [unwired: 2 in, 3 out]
      }
      event "三级过滤系统": Value Change {
        n168 = event-data() -> ()  [unwired: 1 in, 6 out]
        n169 = Build Array("三级过滤系统") -> (w316:bool[])
        n170 = Bundle By Name(cluster=T13 {"命令"="线圈写入", "data"={"starting address"=2802, "coil values"=[]}} ("元素"), "data.coil values"=w316) -> (w320:T13)
        n171 = Flush Queue(queue=w318) -> (queue out=w319:refnum<queue>)  [unwired: 1 in, 2 out]
        n172 = Enqueue Element At Opposite End(queue=w319, element=w320) -> ()  [unwired: 2 in, 3 out]
      }
      event "更新程序": Value Change {
        n173 = event-data() -> ("NewVal"=w322:bool)  [unwired: 1 in, 5 out]
        n174 = case shown="真" w322 {
          tunnel: [cluster{"命令":string, "数据":variant} {"命令"="init", "数据"=variant} ("元素") w329] -> w324
          frame False {
          }
          frame True {
            n175 = Two Button Dialog(message="警告，非专业人士请勿进行此操作！！！\n请确认是否继续？" ("消息")) -> (T button?=w328:bool)  [unwired: 2 in]
            n176 = case shown="假" w328 {
              tunnel: [_ cluster{"命令":string, "数据":variant} {"命令"="shutdown", "数据"=variant} ("元素")] -> w329
              frame False {
                n177 = local write "更新程序"(FALSE ("释放串口")) -> ()
              }
              frame True {
              }
            }
          }
        }
        n178 = Flush Queue(queue=w325) -> (queue out=w323:refnum<queue>)  [unwired: 1 in, 2 out]
        n179 = Enqueue Element(queue=w323, element=w324) -> ()  [unwired: 2 in, 3 out]
      }
    }
  }
  n180 = vi-ref "PLC.lvlib:断电保存变量.vi"() -> (w9:refnum<vi>)
  n181 = Obtain Queue(name (unnamed)="采配水" ("名称（未命名）"), element data type=cluster{"命令":string, "数据":variant} {"命令"="", "数据"=variant}) -> (queue out=w21:refnum<queue>, error out=w20:errorcluster)  [unwired: 3 in, 1 out]
  n182 = call <userlib>:"Read Panel from INI__ogtk.vi"("error in (no error)"=w8, "VI ref"=w9, "refnum"=w2) -> ("error out"=w11:errorcluster, "refnum out"=w10:T5)  [unwired: 7 in]
  n183 = property on="多列列表框" class="MCListbox (严格)"("ItemNames"=string[][] [["待机"], ["初始化"], ["流通池润洗"], ["沉淀池润洗"], ["采样"], ["沉淀"], ["氨氮水样池进样"], ["配水"], ["外部管路反冲洗"], ["内部管路反冲洗"], ["流通池储水"], ["结束"]] ("项名")) -> ()  [unwired: 2 in, 2 out]
  n184 = call <vilib>:"Close Config Data.vi"("error in (no error)"=w11, "refnum"=w10) -> ("error out"=w1:errorcluster)  [unwired: 8 in, 1 out]
  n185 = Enqueue Element(queue=w21, element=cluster{"命令":string, "数据":variant} {"命令"="init", "数据"=variant} ("元素"), error in (no error)=w20) -> (queue out=w16:refnum<queue>, error out=w18:errorcluster)  [unwired: 1 in, 1 out]
  n186 = while {
    tunnel: w16 -> [w337]
    tunnel: w18 -> [w336]
    shift-right: [w339] -> w15
    shift-left: refnum<class "MB_Master.lvclass"> refnum ("MB session out") -> [w338]
    shift-right: [w334] -> w12
    shift-left: errorcluster {"status"=FALSE, "code"=0, "source"=""} ("error out") -> [w333]
    tunnel: w1 -> [_]
    stop <- FALSE stop-if-true
    n187 = case shown="无错误" w333 {
      selector: w333 -> [w347 w487]
      tunnel: [w349 w484] -> w339
      tunnel: w338 -> [w348 w485]
      tunnel: [w341 w488] -> w334
      tunnel: w337 -> [w344 w491]
      tunnel: w336 -> [w343 _]
      tunnel: [w345 _] -> _
      tunnel: [w340 TRUE ("status")] -> w332
      frame No Error {
        n188 = Dequeue Element(queue=w344, error in (no error)=w343) -> (element=w342:cluster{"命令":string, "数据":variant})  [unwired: 1 in, 3 out]
        n189 = Unbundle By Name(w342) -> ("命令"=w346:string)
        n190 = case shown="\"读状态\"" w346 {
          tunnel: [w351 w352 w376 w425 w437 w447 w457 w470] -> w349
          tunnel: w348 -> [w351 w365 w403 w430 w440 w450 w460 w470]
          tunnel: [w350 w362 w372 w424 w438 w448 w458 w461] -> w341
          tunnel: w347 -> [w350 w367 w406 w429 w439 w449 w459 w466]
          tunnel: [_ _ _ _ _ _ _ TRUE] -> w345
          tunnel: w342 -> [_ _ _ _ w436 w446 w456 _]
          frame "idle", Default {
          }
          frame "init" {
            n191 = call-dynamic "Close Session.vi"("error in (no error)"=w367, "MB session in"=w365) -> ("error out"=w366:errorcluster)  [unwired: 9 in]
            n192 = call <vilib>:"Clear Errors.vi"("error in (no error)"=w366) -> ("error out"=w354:errorcluster)  [unwired: 5 in, 1 out]
            n193 = TCP Open Connection(address="192.168.1.200" ("IP Address"), remote port or service name=u16 502 ("远程端口或服务名称"), error in (no error)=w354) -> (connection ID=w356:refnum<k5>, error out=w355:errorcluster)  [unwired: 2 in]
            n194 = TCP Write(connection ID=w356, data in="\u0002004701R04047560A5B\u0003" ("写入缓冲区"), error in (no error)=w355) -> (connection ID out=w357:refnum<k5>, error out=w358:errorcluster)  [unwired: 1 in, 1 out]
            n195 = TCP Close Connection(connection ID=w357, error in (no error)=w358) -> (error out=w353:errorcluster)  [unwired: 1 in, 1 out]
            n196 = call <vilib>:"Open TCP Session.vi"("Slave ID (255)"=u8 10, "error in (no error)"=w353, "IP Address"="192.168.1.200") -> ("error out"=w362:errorcluster, "MB_TCP session"=w352:refnum<class "MB_Master_TCP.lvclass">)  [unwired: 7 in]
            n197 = global write "采配水全局变量.vi" "Pump MB session in"(w352) -> ()
          }
          frame "读状态" {
            n198 = call <vilib>:"Read Holding Registers.vi"("error in (no error)"=w406, "quantity"=u16 40 ("number of holding registers"), "starting address"=u16 0, "MB session in"=w403) -> ("error out"=w369:errorcluster, "Registers"=w385:u16[], "MB session out"=w384:refnum<class "MB_Master.lvclass">)  [unwired: 5 in]
            "状态" <- w385
            n199 = case shown="无错误" w369 {
              tunnel: w385 -> [w418 _]
              frame No Error {
                n200 = Array To Cluster(array=w418) -> (cluster=w417:T19)
                n201 = Array Subset(array=w418, index=20 ("索引")) -> (w421:u16[])  [unwired: 1 in]
                n202 = global write "采配水全局变量.vi" "状态"(w417) -> ()
                n203 = call "FATEK_HexToString.vi"("数组"=w421) -> ("STRING"=w420:string[])  [unwired: 10 in]
                n204 = Index Array(array=w420) -> (element=→"采配水版本号":string)  [unwired: 1 in]
              }
              frame Error {
              }
            }
            n205 = call <vilib>:"Read Holding Registers.vi"("error in (no error)"=w369, "quantity"=u16 32, "starting address"=u16 200, "MB session in"=w384) -> ("error out"=w383:errorcluster, "Registers"=w379:u16[], "MB session out"=w382:refnum<class "MB_Master.lvclass">)  [unwired: 5 in]
            n206 = Array To Cluster(array=w379) -> (cluster=w378:T20)
            n207 = global write "采配水全局变量.vi" "工作计时"(w378) -> ()
            n208 = call <vilib>:"Read Holding Registers.vi"("error in (no error)"=w383, "quantity"=u16 6 ("number of holding registers"), "starting address"=u16 3840, "MB session in"=w382) -> ("error out"=w368:errorcluster, "Registers"=w386:u16[], "MB session out"=w400:refnum<class "MB_Master.lvclass">)  [unwired: 5 in]
            n209 = case shown="无错误" w368 {
              tunnel: w386 -> [w412 _]
              frame No Error {
                n210 = Array To Cluster(array=w412) -> (cluster=w413:T21)
                n211 = global write "采配水全局变量.vi" "AD"(w413) -> ()
                n212 = global read "断电保存变量.vi" "AD线性关系"() -> (w411:T22)
                n213 = To Word Integer(number=w412) -> (16bit integer=w410:i16[])
                n214 = for {
                  tunnel: w411 -> [w416] mode=indexing
                  tunnel: w410 -> [w415] mode=indexing
                  tunnel: [w414] -> w409 mode=indexing
                  n215 = call "线性转换.vi"("线性关系"=w416, "input"=w415) -> ("output"=w414:dbl)  [unwired: 9 in]
                }
                n216 = Array To Cluster(array=w409) -> (cluster=w408:T23)
                n217 = Unbundle By Name(w408) -> ("[2]"=→"过滤压力":dbl)
                n218 = global write "采配水全局变量.vi" "转换值"(w408) -> ()
              }
              frame Error {
              }
            }
            n219 = call <vilib>:"Read Coils.vi"("error in (no error)"=w368, "quantity"=u16 32 ("number of coils"), "starting address"=u16 0, "MB session in"=w400) -> ("error out"=w396:errorcluster, "Coils"=w387:bool[], "MB session out"=w397:refnum<class "MB_Master.lvclass">)  [unwired: 5 in]
            n220 = global write "采配水全局变量.vi" "输出状态"(w387) -> ()
            n221 = call <vilib>:"Read Coils.vi"("error in (no error)"=w396, "quantity"=u16 16 ("number of coils"), "starting address"=u16 1000, "MB session in"=w397) -> ("error out"=w392:errorcluster, "Coils"=w388:bool[], "MB session out"=w393:refnum<class "MB_Master.lvclass">)  [unwired: 5 in]
            n222 = global write "采配水全局变量.vi" "输入状态"(w388) -> ()
            n223 = call <vilib>:"Read Coils.vi"("error in (no error)"=w392, "quantity"=u16 16 ("number of coils"), "starting address"=u16 2500, "MB session in"=w393) -> ("error out"=w375:errorcluster, "Coils"=w389:bool[], "MB session out"=w377:refnum<class "MB_Master.lvclass">)  [unwired: 5 in]
            n224 = global write "采配水全局变量.vi" "报警簇"(w389) -> ()
            n225 = call <vilib>:"Read Coils.vi"("error in (no error)"=w375, "quantity"=u16 1 ("starting address"), "starting address"=u16 2802, "MB session in"=w377) -> ("error out"=w372:errorcluster, "Coils"=w371:bool[], "MB session out"=w376:refnum<class "MB_Master.lvclass">)  [unwired: 5 in]
            n226 = Index Array(array=w371) -> (element=w370:bool)  [unwired: 1 in]
            n227 = local write "三级过滤系统"(w370) -> ()
          }
          frame "读参数" {
            n228 = call <vilib>:"Read Holding Registers.vi"("error in (no error)"=w429, "quantity"=u16 24 ("number of holding registers"), "starting address"=u16 100, "MB session in"=w430) -> ("error out"=w424:errorcluster, "Registers"=w426:u16[], "MB session out"=w425:refnum<class "MB_Master.lvclass">)  [unwired: 5 in]
            n229 = Array To Cluster(array=w426) -> (cluster=w423:T24)
            n230 = global write "采配水全局变量.vi" "参数设置"(w423) -> ()
          }
          frame "多个写入" {
            n231 = Unbundle By Name(w436) -> ("数据"=w435:variant)
            n232 = Variant To Data(type=T16 {"starting address"=0, "holding register values"=[]}, Variant=w435) -> (data=w433:T16)  [unwired: 1 in, 1 out]
            n233 = Unbundle By Name(w433) -> ("starting address"=w432:u16, "holding register values"=w431:u16[])
            n234 = call <vilib>:"Write Multiple Registers.vi"("error in (no error)"=w439, "values"=w431, "starting address"=w432, "MB session in"=w440) -> ("error out"=w438:errorcluster, "MB session out"=w437:refnum<class "MB_Master.lvclass">)  [unwired: 6 in]
          }
          frame "单个写入" {
            n235 = Unbundle By Name(w446) -> ("数据"=w445:variant)
            n236 = Variant To Data(type=T17 {"starting address"=0, "holding register value"=0}, Variant=w445) -> (data=w443:T17)  [unwired: 1 in, 1 out]
            n237 = Unbundle By Name(w443) -> ("starting address"=w442:u16, "holding register value"=w441:u16)
            n238 = call <vilib>:"Write Single Register.vi"("error in (no error)"=w449, "value"=w441, "address"=w442, "MB session in"=w450) -> ("error out"=w448:errorcluster, "MB session out"=w447:refnum<class "MB_Master.lvclass">)  [unwired: 6 in]
          }
          frame "线圈写入" {
            n239 = Unbundle By Name(w456) -> ("数据"=w455:variant)
            n240 = Variant To Data(type=T18 {"starting address"=0, "coil values"=[]}, Variant=w455) -> (data=w453:T18)  [unwired: 1 in, 1 out]
            n241 = Unbundle By Name(w453) -> ("starting address"=w452:u16, "coil values"=w451:bool[])
            n242 = call <vilib>:"Write Multiple Coils.vi"("error in (no error)"=w459, "values"=w451, "starting address"=w452, "MB session in"=w460) -> ("error out"=w458:errorcluster, "MB session out"=w457:refnum<class "MB_Master.lvclass">)  [unwired: 6 in]
          }
          frame "shutdown" {
            n243 = call <vilib>:"Write Single Register.vi"("error in (no error)"=w466, "value"=u16 0, "address"=u16 4047, "MB session in"=w470) -> ("error out"=w465:errorcluster, "MB session out"=w469:refnum<class "MB_Master.lvclass">)  [unwired: 6 in]
            n244 = call-dynamic "Close Session.vi"("error in (no error)"=w465, "MB session in"=w469) -> ("error out"=w471:errorcluster)  [unwired: 9 in]
            n245 = call "文件对话框"("start path"=path "D:/SRC") -> ("selected path"=w464:path, "cancelled"=w462:bool)  [unwired: 11 in, 2 out]
            n246 = call <vilib>:"Clear Errors.vi"("error in (no error)"=w471) -> ("error out"=w461:errorcluster)  [unwired: 5 in, 1 out]
            n247 = case shown="假" w462 {
              tunnel: w464 -> [w477 _]
              tunnel: w461 -> [_ _]
              frame False {
                n248 = Path To String(path=w477) -> (string=w474:string)
                n249 = Format Into String(format string="  - \"%s\"" ("格式字符串"), initial string="\"C:\\Program Files\\Fatek\\WinProladder\\WProlad.exe\"" ("command line"), w474) -> (resulting string=w475:string)  [unwired: 1 in, 1 out]
                n250 = call <vilib>:"System Exec.vi"("command line"=w475) -> ("error out"=w478:errorcluster)  [unwired: 7 in, 3 out]
                n251 = case shown="错误" w478 {
                  tunnel: w474 -> [_ w481]
                  frame No Error {
                  }
                  frame Error {
                    n252 = Format Into String(format string="  - \"%s\"" ("格式字符串"), initial string="\"C:\\Program Files (x86)\\Fatek\\WinProladder\\WProlad.exe\"" ("command line"), w481) -> (resulting string=w479:string)  [unwired: 1 in, 1 out]
                    n253 = call <vilib>:"System Exec.vi"("command line"=w479) -> ()  [unwired: 7 in, 4 out]
                  }
                }
              }
              frame True {
              }
            }
          }
        }
        n254 = Unbundle By Name(w341) -> ("status"=w340:bool)
      }
      frame Error {
        n255 = property class="MB_Master"(reference=w485) -> (reference out=w484:refnum<class "MB_Master.lvclass">, "Properties:Session Valid"=w486:bool)  [unwired: 1 in, 1 out]
        n256 = Flush Queue(queue=w491) -> (queue out=w490:refnum<queue>)  [unwired: 1 in, 2 out]
        n257 = Wait (ms)(milliseconds to wait=u32 2000 ("等待时间（毫秒）")) -> ()  [unwired: 1 out]
        n258 = case shown="假" w486 {
          tunnel: w490 -> [w493 _]
          frame False {
            n259 = Enqueue Element At Opposite End(queue=w493, element=cluster{"命令":string, "数据":variant} {"命令"="init", "数据"=variant} ("元素")) -> ()  [unwired: 2 in, 3 out]
          }
          frame True {
          }
        }
        n260 = call <vilib>:"Clear Errors.vi"("error in (no error)"=w487) -> ("error out"=w488:errorcluster)  [unwired: 5 in, 1 out]
      }
    }
    "通讯故障" <- w332
    n261 = global write "采配水全局变量.vi" "通讯故障"(w332) -> ()
  }
  n262 = call-dynamic "Close Session.vi"("error in (no error)"=w12, "MB session in"=w15) -> ()  [unwired: 9 in, 1 out]
